vi "nanocal -- nuclear schottky fit V8.vi"() -> ()   [LabVIEW 2021]
uses:
  filename-pattern.ctl
  show-win- control.ctl
  cursor winow.ctl
  nanocal_data_read_format.ctl
  3-lorentzian-parameters.ctl
  nameformattingitem.ctl
  nanocal_side_selector.ctl
  filename-action.ctl
  nanocal -- gradient descent -- parameters.ctl
  linear regression type.ctl
  nanocal-goodness-weighting-strategy.ctl
  3D curvature triplet control -- V2.ctl
  cursor window action.ctl
  cursor action.ctl
  2Dwindow.ctl
  3-lorentzian-heat-response action.ctl
  publisher action.ctl
  <vilib>/Utility/miscctls.llb/LVMapReplaceAction.ctl
  nanocal -- gradient descent -- action.ctl
  array action.ctl
  cursor sate.ctl
  interpolation state - real.ctl
  agregator -- action.ctl
  mathematica string map action.ctl
  nanocal -- defaut parameter manager action-- V1.ctl
  nanocal -- plotstring file action.ctl
  file -- read-write control.ctl
  array -- freq-voltage transformations action.ctl
  nanocal_raw_file_manage_action_V1.ctl
  KM_file -- read-write control.ctl
  replace cursor action stack.vi
  Q -- range multiplier -- real -- V2.vi
  Q - not nan and gtr than zero - Real.vi
  Q - not nan -- real.vi
  Q -- check range -- i -- real.vi
  array - smart min max.vi
  3-lorentzian-heat-response -- V4.vi/142dd4c5-f9ed-c64b-bc14-a88e3e2c450a.vi
  nanocal -- tensors and stuff -- V1.vi
  nanocal -- nuclear schottky goodness V6.vi
  linear interpolation - real -- V2.vi
  <vilib>/AdvancedString/Delimited String to 1D String Array.vi
  array -- freq-voltage transformations.vi/05c44075-957c-bc42-b6fa-2799d0bc0485.vi
  tale of three indices.vi
  filter -- window span logic.vi
  linear interp iiii- complex - z-omega - divide.vi
  linear interpolation iiii- complex.vi
  containing bix.vi
  array -- 3-finitediff.vi
  5-lorentzian-heat-response -- analytic derivatives -- grad and curvature -- V6.vi
  <vilib>/Array/Sort 2D Array - Pop Stack.vi
  <vilib>/Array/Sort 2D Array - Push Stack.vi
  array -- freq-voltage transformations.vi/05c44075-957c-bc42-b6fa-2799d0bc0485.vi/269d4b3b-47f5-49e3-8884-44851e4dd9d5.vi
  array -- freq-voltage transformations.vi/05c44075-957c-bc42-b6fa-2799d0bc0485.vi/6d99389c-673d-4efb-bf33-19b32bcf4cf8.vi
  command stack.vi
  tale of three indices -- check state.vi
  Q -- check range -- i -- integer.vi
  linear interp iiii- complex - z-omega.vi
  line -- complex.vi
  Q - not nan -- integer.vi
  <vilib>/Analysis/baseanly.llb/A x B.vi
  <vilib>/Analysis/baseanly.llb/Complex A x B.vi
  <vilib>/Analysis/Matrix/Numeric/Conversions/Array To Matrix.vi
  <vilib>/Analysis/Matrix/Numeric/Conversions/Array To Matrix - RA2.vi
  <vilib>/Analysis/baseanly.llb/Inverse Matrix.vi
  <vilib>/Analysis/baseanly.llb/Real Inverse Matrix.vi
  <vilib>/Analysis/Matrix/Numeric/Conversions/Matrix To Array.vi
  <vilib>/Analysis/Matrix/Numeric/Conversions/Matrix To Array - RM.vi
  <vilib>/Analysis/Matrix/Numeric/Conversions/Array To Matrix - RA.vi
  <vilib>/Analysis/7linalg.llb/Solve Linear Equations.vi
  <vilib>/Analysis/7linalg.llb/Solve Linear Equations (multiple right hand).vi
  <vilib>/Analysis/polynomials.llb/Polynomial Roots.vi
  <vilib>/Analysis/polynomials.llb/Polynomial Roots (DBL).vi
  <vilib>/Comparison/Less/Less Functor/Less Functor.lvclass
panel:
  in  "tab 8":enum32{"main", "energy profile", "internals"}(tab)
  in  "D. data & fit":enum32{"main"}(tab)
  out "Plot: circles":cluster{"Freq out (Hz)":dbl[], dbl[]}[](graph)
  in  "scale gauge: Plot: circles":dbl(slide)=743510538.726018 min=0.0 max=0.3 step=1e-06 scale=1000000.0..10000000000.0 scale format="%#_3p"
  in  "ω0 (rad/sec)":dbl(slide)=14.871166449464935 scale=0.001..50000.0 scale format="%#_2p"
  in  "E. parameters & open /save":enum32{"logarithmic derivatives"}(tab)
  out "vector of dG/dlogα":dbl[](array[numeric])=[1.7883295749176973, 3.668532274452499, -8.457041272332772, -0.30777115676432043, -0.9594535744754293, -49.05782552987492] format="%#_2f"
  in  "factors":cluster{"scaling":dbl, "what":T1}[](array[cluster])=[{"scaling"=1.0, "what"=enum."ζ"}, {"scaling"=1.0, "what"=enum."τ1"}, {"scaling"=1.0, "what"=enum."τS"}, {"scaling"=1.0, "what"=enum."τN"}, {"scaling"=1.0, "what"=enum."τC"}, {"scaling"=1.0, "what"=enum."κ0"}]
  in  "tab77":enum32{"Page 1"}(tab)
  in  "τC":dbl(slide)=0.001657645209 min=0.0 max=0.3 step=1e-06 scale=0.0001..1.0 scale format="%#_3p"
  in  "τN":dbl(slide)=0.017176281362 min=0.0 max=0.3 step=1e-06 scale=1e-06..1.0 scale format="%#_3p"
  in  "τS":dbl(slide)=0.023837806105 min=0.0 max=0.3 step=1e-06 scale=0.0001..1.0 scale format="%#_3p"
  in  "ζ":dbl(slide)=0.068889386962 min=0.0 max=0.3 step=1e-06 scale=1e-05..1.0 scale format="%#_3p"
  in  "T1":dbl(slide)=0.042189760597 min=0.0 max=0.3 step=1e-06 scale=0.0001..1.0 scale format="%#_3p"
  in  "κ0":dbl(slide)=1.746e-09 min=0.0 max=0.3 step=1e-12 scale=1e-10..1e-06 scale format="%#_3p"
  in  "newton parameters":T2={"method"=enum."newton", "weighting"=enum."dω |dz/dω|", "PID-P"=0.16017985150009284, "PID-I"=3} {"PID-P" scale=1e-09..10.0 scale format="%#_3p"}
  in  "tab 4":enum32{"Page 1"}(tab)
  in  "go / pause!":bool
  in  "tab 7":enum32{"Page 1"}(tab)
  in  "tab 3":enum32{"Page 1"}(tab)
  out "key":string="IDS0187_210310_RAW_cal__ref_"
  out "T (K)":dbl=0.3 format="%#_3f"
  out "θ (deg)":dbl=90.0 format="%#_3f"
  out "B (T)":dbl=12.0 format="%#_3f"
  in  "tab 6":enum32{"Page 1"}(tab)
  in  "τ→Math! :p":bool
  in  "selection :|\\":u16(ring)=5 caption="files" items=["IDS0183_210310_RAW_cal_CeCoIn5_2nd_071_12T_0.120K_90deg_Tdep_raw_.dat", "IDS0184_210310_RAW_cal_CeCoIn5_2nd_072_12T_0.148K_90deg_Tdep_raw_.dat", "IDS0181_210310_RAW_cal_CeCoIn5_2nd_070_12T_0.179K_90deg_fsweep_Tdep_raw_.dat", "IDS0185_210310_RAW_cal_CeCoIn5_2nd_073_12T_0.197K_90deg_Tdep_raw_.dat", "IDS0186_210310_RAW_cal_CeCoIn5_2nd_074_12T_0.249K_90deg_Tdep_raw_.dat", "IDS0187_210310_RAW_cal_CeCoIn5_2nd_075_12T_0.300K_90deg_Tdep_raw_.dat", "IDS0188_210310_RAW_cal_CeCoIn5_2nd_076_12T_0.360K_90deg_Tdep_raw_.dat", "IDS0189_210310_RAW_cal_CeCoIn5_2nd_077_12T_0.430K_90deg_Tdep_raw_.dat", "IDS0190_210310_RAW_cal_CeCoIn5_2nd_078_12T_0.512K_90deg_Tdep_raw_.dat", "IDS0191_210310_RAW_cal_CeCoIn5_2nd_079_12T_0.610K_90deg_Tdep_raw_.dat", "IDS0192_210310_RAW_cal_CeCoIn5_2nd_080_12T_0.810K_90deg_Tdep_raw_.dat", "IDS0193_210310_RAW_cal_CeCoIn5_2nd_081_12T_1.1K_90deg_Tdep_raw_.dat", "IDS0194_210310_RAW_cal_CeCoIn5_2nd_082_12T_1.8K_90deg_Tdep_raw_.dat", "IDS0195_210310_RAW_cal_CeCoIn5_2nd_083_12T_3.0K_90deg_Tdep_raw_.dat", "IDS0196_210310_RAW_cal_CeCoIn5_2nd_084_12T_5.7K_90deg_Tdep_raw_.dat"]
  in  "tab 5":enum32{"Page 1"}(tab)
  in  "Math→τ! :q":bool
  in  "tab 44":enum32{"default values "}(tab)
  in  "defaults selector":T5(array[cluster])=[{"Plost: sweep window"=enum."ζ", "used default"=FALSE}, {"Plost: sweep window"=enum."noiseT", "used default"=TRUE}, {"Plost: sweep window"=enum."τS", "used default"=FALSE}, {"Plost: sweep window"=enum."τN", "used default"=FALSE}, {"Plost: sweep window"=enum."τC", "used default"=FALSE}, {"Plost: sweep window"=enum."Re(offset)", "used default"=TRUE}]
  in  "default values string":string="<| \"0\"->   <|\"T\" -> 0.12, \"Reoff\"-> -130000000.0|>,\n\"1\"->   <|\"T\" -> 0.15, \"Reoff\"-> -70000000.0|>,\n\"2\"->   <|\"T\" -> 0.17, \"Reoff\"-> -50000000.0|>,\n\"3\"->   <|\"T\" -> 0.20, \"Reoff\"-> -28000000.0|>,\n\"4\"->   <|\"T\" -> 0.25, \"Reoff\"-> -14000000.0|>,\n\"5\"->   <|\"T\" -> 0.30, \"Reoff\"-> -8000000.0|>,\n\"6\"->   <|\"T\" -> 0.36, \"Reoff\"-> -4500000.0|>,\n\"7\"->   <|\"T\" -> 0.43, \"Reoff\"-> -3000000.0|>,\n\"8\"->   <|\"T\" -> 0.51, \"Reoff\"-> -2500000.0|>,\n\"9\"->   <|\"T\" -> 0.61, \"Reoff\"-> -1000000.0|>,\n\"10\"->  <|\"T\" -> 0.81, \"Reoff\"-> -700000.0|>,\n\"11\"->  <|\"T\" -> 1.1, \"Reoff\"-> -600000.0|>,\n\"12\"->  <|\"T\" -> 1.8, \"Reoff\"-> -250000.0|>,\n\"13\"->  <|\"T\" -> 3.0, \"Reoff\"-> -130000.0|>,\n\"14\"->  <|\"T\" -> 5.7, \"Reoff\"-> -50000.0|>\n|>\n"
  in  "load defaults":bool
  in  "F. plots & stuff":enum32{"Page 1"}(tab)
  in  "X selector":T1=enum."T (K)"
  in  "Plot:  colors":cluster{"Freq out (Hz)":dbl[], dbl[]}[](graph)=[{"Freq out (Hz)"=[0.12, 0.148, 0.179, 0.197, 0.249, 0.3, 0.36, 0.43, 0.512, 0.61, 0.81, 1.1, 1.8, 3.0, 5.7], [0.375235391174, 0.267189614091, 0.199306617611, 0.169435500052, 0.10023219366, 0.068889386962, 0.050855621628, 0.038379394547, 0.030757711173, 0.024472356387, 0.019125590894, 0.016340595254, 0.01263439258, 0.019026086981, 0.019858524497]}, {"Freq out (Hz)"=[0.12, 0.148, 0.179, 0.197, 0.249, 0.3, 0.36, 0.43, 0.512, 0.61, 0.81, 1.1, 1.8, 3.0, 5.7], [0.100390183494, 0.086925369127, 0.070107577087, 0.06552222252, 0.0499817149, 0.042189760597, 0.035114064267, 0.030049345911, 0.024931554661, 0.022407083343, 0.016432131318, 0.01691523202, 0.012311180561, 0.018297259133, 0.012821278093]}, {"Freq out (Hz)"=[0.12, 0.148, 0.179, 0.197, 0.249, 0.3, 0.36, 0.43, 0.512, 0.61, 0.81, 1.1, 1.8, 3.0, 5.7], [0.059883674441, 0.044416499058, 0.034354681127, 0.031885966152, 0.026964705596, 0.023837806105, 0.021745076003, 0.020197203084, 0.019059366283, 0.017600386438, 0.016139955363, 0.015114072822, 0.011880374999, 0.007367031681, 0.004631070276]}, {"Freq out (Hz)"=[0.12, 0.148, 0.179, 0.197, 0.249, 0.3, 0.36, 0.43, 0.512, 0.61, 0.81, 1.1, 1.8, 3.0, 5.7], [0.583268417564, 0.254096954422, 0.115326183519, 0.085736532349, 0.034498560244, 0.017176281362, 0.009940720882, 0.005279271749, 0.002804912424, 0.001730254025, 0.000695948251, 0.000265648688, 6.6834392e-05, 1.2328467e-05, 1.621029e-06]}, {"Freq out (Hz)"=[0.12, 0.148, 0.179, 0.197, 0.249, 0.3, 0.36, 0.43, 0.512, 0.61, 0.81, 1.1, 1.8, 3.0, 5.7], [0.00101538821, 0.000963914391, 0.001029913549, 0.00108551185, 0.001422553924, 0.001657645209, 0.002035754152, 0.002296433055, 0.00240095569, 0.003444856237, 0.003787605771, 0.003610389555, 0.00409358538, 0.005085235141, 0.003887972994]}, {"Freq out (Hz)"=[], [0.12, 0.13, 0.14, 0.15000000000000002, 0.16000000000000003, 0.17000000000000004, 0.18000000000000005, 0.19000000000000006, 0.20000000000000007, 0.21000000000000008, 0.22000000000000008, 0.2300000000000001, 0.2400000000000001, 0.2500000000000001, 0.2600000000000001, 0.27000000000000013, 0.28000000000000014, 0.29000000000000015, 0.30000000000000016, 0.31000000000000016, 0.3200000000000002, 0.3300000000000002, 0.3400000000000002, 0.3500000000000002, 0.3600000000000002, 0.3700000000000002, 0.3800000000000002, 0.39000000000000024, 0.40000000000000024, 0.41000000000000025, 0.42000000000000026, 0.43000000000000027, 0.4400000000000003, 0.4500000000000003, 0.4600000000000003, 0.4700000000000003, 0.4800000000000003, 0.4900000000000003, 0.5000000000000003, 0.5100000000000003, 0.5200000000000004, 0.5300000000000004, 0.5400000000000004, 0.5500000000000004, 0.5600000000000004, 0.5700000000000004, 0.5800000000000004, 0.5900000000000004, 0.6000000000000004, 0.6100000000000004, 0.6200000000000004, 0.6300000000000004, 0.6400000000000005, 0.6500000000000005, 0.6600000000000005, 0.6700000000000005, 0.6800000000000005, 0.6900000000000005, 0.7000000000000005, 0.7100000000000005, 0.7200000000000005, 0.7300000000000005, 0.7400000000000005, 0.7500000000000006, 0.7600000000000006, 0.7700000000000006, 0.7800000000000006, 0.7900000000000006, 0.8000000000000006, 0.8100000000000006, 0.8200000000000006, 0.8300000000000006, 0.8400000000000006, 0.8500000000000006, 0.8600000000000007, 0.8700000000000007, 0.8800000000000007, 0.8900000000000007, 0.9000000000000007, 0.9100000000000007, 0.9200000000000007, 0.9300000000000007, 0.9400000000000007, 0.9500000000000007, 0.9600000000000007, 0.9700000000000008, 0.9800000000000008, 0.9900000000000008, 1.0000000000000009, 1.0100000000000007, 1.020000000000001, 1.0300000000000007, 1.040000000000001, 1.0500000000000007, 1.060000000000001, 1.0700000000000007, 1.080000000000001, 1.0900000000000007, 1.100000000000001, 1.1100000000000008, 1.120000000000001, 1.1300000000000008, 1.140000000000001, 1.1500000000000008, 1.160000000000001, 1.1700000000000008, 1.180000000000001, 1.1900000000000008, 1.200000000000001, 1.2100000000000009, 1.220000000000001, 1.2300000000000009, 1.240000000000001, 1.2500000000000009, 1.2600000000000011, 1.270000000000001, 1.2800000000000011, 1.290000000000001, 1.3000000000000012, 1.310000000000001, 1.3200000000000012, 1.330000000000001, 1.3400000000000012, 1.350000000000001, 1.3600000000000012, 1.370000000000001, 1.3800000000000012, 1.390000000000001, 1.4000000000000012, 1.410000000000001, 1.4200000000000013, 1.430000000000001, 1.4400000000000013, 1.450000000000001, 1.4600000000000013, 1.470000000000001, 1.4800000000000013, 1.490000000000001, 1.5000000000000013, 1.5100000000000011, 1.5200000000000014, 1.5300000000000011, 1.5400000000000014, 1.5500000000000012, 1.5600000000000014, 1.5700000000000012, 1.5800000000000014, 1.5900000000000012, 1.6000000000000014, 1.6100000000000012, 1.6200000000000014, 1.6300000000000012, 1.6400000000000015, 1.6500000000000012, 1.6600000000000015, 1.6700000000000013, 1.6800000000000015, 1.6900000000000013, 1.7000000000000015, 1.7100000000000013, 1.7200000000000015, 1.7300000000000013, 1.7400000000000015, 1.7500000000000013, 1.7600000000000016, 1.7700000000000014, 1.7800000000000016, 1.7900000000000014, 1.8000000000000016, 1.8100000000000014, 1.8200000000000016, 1.8300000000000014, 1.8400000000000016, 1.8500000000000014, 1.8600000000000017, 1.8700000000000014, 1.8800000000000017, 1.8900000000000015, 1.9000000000000017, 1.9100000000000015, 1.9200000000000017, 1.9300000000000015, 1.9400000000000017, 1.9500000000000015, 1.9600000000000017, 1.9700000000000015, 1.9800000000000018, 1.9900000000000015, 2.0000000000000018, 2.0100000000000016, 2.020000000000002, 2.0300000000000016, 2.040000000000002, 2.0500000000000016, 2.060000000000002, 2.0700000000000016, 2.080000000000002, 2.0900000000000016, 2.100000000000002, 2.1100000000000017, 2.120000000000002, 2.1300000000000017, 2.140000000000002, 2.150000000000002, 2.160000000000002, 2.1700000000000017, 2.180000000000002, 2.190000000000002, 2.200000000000002, 2.2100000000000017, 2.220000000000002, 2.230000000000002, 2.240000000000002, 2.2500000000000018, 2.260000000000002, 2.2700000000000022, 2.280000000000002, 2.290000000000002, 2.300000000000002, 2.3100000000000023, 2.320000000000002, 2.330000000000002, 2.340000000000002, 2.3500000000000023, 2.360000000000002, 2.370000000000002, 2.380000000000002, 2.3900000000000023, 2.400000000000002, 2.410000000000002, 2.420000000000002, 2.4300000000000024, 2.440000000000002, 2.450000000000002, 2.460000000000002, 2.4700000000000024, 2.480000000000002, 2.490000000000002, 2.500000000000002, 2.5100000000000025, 2.5200000000000022, 2.530000000000002, 2.5400000000000023, 2.5500000000000025, 2.5600000000000023, 2.570000000000002, 2.5800000000000023, 2.5900000000000025, 2.6000000000000023, 2.610000000000002, 2.6200000000000023, 2.6300000000000026, 2.6400000000000023, 2.650000000000002, 2.6600000000000024, 2.6700000000000026, 2.6800000000000024, 2.690000000000002, 2.7000000000000024, 2.7100000000000026, 2.7200000000000024, 2.730000000000002, 2.7400000000000024, 2.7500000000000027, 2.7600000000000025, 2.7700000000000022, 2.7800000000000025, 2.7900000000000027, 2.8000000000000025, 2.8100000000000023, 2.8200000000000025, 2.8300000000000027, 2.8400000000000025, 2.8500000000000023, 2.8600000000000025, 2.8700000000000028, 2.8800000000000026, 2.8900000000000023, 2.9000000000000026, 2.910000000000003, 2.9200000000000026, 2.9300000000000024, 2.9400000000000026, 2.950000000000003, 2.9600000000000026, 2.9700000000000024, 2.9800000000000026, 2.990000000000003, 3.0000000000000027, 3.0100000000000025, 3.0200000000000027, 3.030000000000003, 3.0400000000000027, 3.0500000000000025, 3.0600000000000027, 3.070000000000003, 3.0800000000000027, 3.0900000000000025, 3.1000000000000028, 3.110000000000003, 3.1200000000000028, 3.1300000000000026, 3.140000000000003, 3.150000000000003, 3.160000000000003, 3.1700000000000026, 3.180000000000003, 3.190000000000003, 3.200000000000003, 3.2100000000000026, 3.220000000000003, 3.230000000000003, 3.240000000000003, 3.2500000000000027, 3.260000000000003, 3.270000000000003, 3.280000000000003, 3.2900000000000027, 3.300000000000003, 3.310000000000003, 3.320000000000003, 3.3300000000000027, 3.340000000000003, 3.350000000000003, 3.360000000000003, 3.3700000000000028, 3.380000000000003, 3.3900000000000032, 3.400000000000003, 3.410000000000003, 3.420000000000003, 3.4300000000000033, 3.440000000000003, 3.450000000000003, 3.460000000000003, 3.4700000000000033, 3.480000000000003, 3.490000000000003, 3.500000000000003, 3.5100000000000033, 3.520000000000003, 3.530000000000003, 3.540000000000003, 3.5500000000000034, 3.560000000000003, 3.570000000000003, 3.580000000000003, 3.5900000000000034, 3.600000000000003, 3.610000000000003, 3.620000000000003, 3.6300000000000034, 3.6400000000000032, 3.650000000000003, 3.6600000000000033, 3.6700000000000035, 3.6800000000000033, 3.690000000000003, 3.7000000000000033, 3.7100000000000035, 3.7200000000000033, 3.730000000000003, 3.7400000000000033, 3.7500000000000036, 3.7600000000000033, 3.770000000000003, 3.7800000000000034, 3.7900000000000036, 3.8000000000000034, 3.810000000000003, 3.8200000000000034, 3.8300000000000036, 3.8400000000000034, 3.850000000000003, 3.8600000000000034, 3.8700000000000037, 3.8800000000000034, 3.8900000000000032, 3.9000000000000035, 3.9100000000000037, 3.9200000000000035, 3.9300000000000033, 3.9400000000000035, 3.9500000000000037, 3.9600000000000035, 3.9700000000000033, 3.9800000000000035, 3.9900000000000038, 4.0000000000000036, 4.010000000000003, 4.020000000000003, 4.030000000000004, 4.040000000000004, 4.050000000000003, 4.060000000000003, 4.070000000000004, 4.080000000000004, 4.090000000000003, 4.100000000000003, 4.110000000000004, 4.120000000000004, 4.1300000000000034, 4.140000000000003, 4.150000000000004, 4.160000000000004, 4.1700000000000035, 4.180000000000004, 4.190000000000004, 4.200000000000004, 4.2100000000000035, 4.220000000000003, 4.230000000000004, 4.240000000000004, 4.2500000000000036, 4.260000000000004, 4.270000000000004, 4.280000000000004, 4.290000000000004, 4.300000000000003, 4.310000000000004, 4.320000000000004, 4.330000000000004, 4.340000000000004, 4.350000000000004, 4.360000000000004, 4.370000000000004, 4.3800000000000034, 4.390000000000004, 4.400000000000004, 4.410000000000004, 4.420000000000004, 4.430000000000004, 4.440000000000004, 4.450000000000004, 4.4600000000000035, 4.470000000000004, 4.480000000000004, 4.490000000000004, 4.500000000000004, 4.510000000000004, 4.520000000000004, 4.530000000000004, 4.540000000000004, 4.550000000000004, 4.560000000000004, 4.570000000000004, 4.5800000000000045, 4.590000000000004, 4.600000000000004, 4.610000000000004, 4.620000000000004, 4.630000000000004, 4.640000000000004, 4.650000000000004, 4.660000000000005, 4.670000000000004, 4.680000000000004, 4.690000000000004, 4.700000000000004, 4.710000000000004, 4.720000000000004, 4.730000000000004, 4.740000000000005, 4.750000000000004, 4.760000000000004, 4.770000000000004, 4.780000000000004, 4.7900000000000045, 4.800000000000004, 4.810000000000004, 4.820000000000005, 4.8300000000000045, 4.840000000000004, 4.850000000000004, 4.860000000000004, 4.8700000000000045, 4.880000000000004, 4.890000000000004, 4.900000000000005, 4.910000000000005, 4.920000000000004, 4.930000000000004, 4.940000000000004, 4.950000000000005, 4.960000000000004, 4.970000000000004, 4.980000000000005, 4.990000000000005, 5.000000000000004, 5.010000000000004, 5.020000000000004, 5.030000000000005, 5.0400000000000045, 5.050000000000004, 5.060000000000005, 5.070000000000005, 5.0800000000000045, 5.090000000000004, 5.100000000000004, 5.110000000000005, 5.1200000000000045, 5.130000000000004, 5.140000000000005, 5.150000000000005, 5.160000000000005, 5.170000000000004, 5.180000000000004, 5.190000000000005, 5.200000000000005, 5.210000000000004, 5.220000000000005, 5.230000000000005, 5.240000000000005, 5.250000000000004, 5.260000000000004, 5.270000000000005, 5.280000000000005, 5.2900000000000045, 5.300000000000005, 5.310000000000005, 5.320000000000005, 5.3300000000000045, 5.340000000000004, 5.350000000000005, 5.360000000000005, 5.3700000000000045, 5.380000000000005, 5.390000000000005, 5.400000000000005, 5.410000000000005, 5.420000000000004, 5.430000000000005, 5.440000000000005, 5.450000000000005, 5.460000000000005, 5.470000000000005, 5.480000000000005, 5.490000000000005, 5.500000000000004, 5.510000000000005, 5.520000000000005, 5.530000000000005, 5.540000000000005, 5.550000000000005, 5.560000000000005, 5.570000000000005, 5.5800000000000045, 5.590000000000005, 5.600000000000005, 5.610000000000005, 5.620000000000005, 5.630000000000005, 5.640000000000005, 5.650000000000005, 5.660000000000005, 5.670000000000005, 5.680000000000005, 5.690000000000005]}]
  in  "what?":T6={"ignore set of !"=TRUE, "set (1T|2B)"=0, "ignore side !"=FALSE, "side (8S|4R)"=0, "ignore θ !"=FALSE, "ignore B !"=FALSE, "T (K)"=1.0, "ignore T !"=TRUE, "θ (∘)"=4.0, "B (T)"=11.0, "lookup"={"set of lookup"={0=1.0, 1=2.0}, "all set of"={1.0, 2.0}, "T lookup"={0=0.12, 1=0.122, 2=0.14, 3=0.148, 4=0.15, 5=0.157, 6=0.16, 7=0.168, 8=0.17, 9=0.178, 10=0.179, 11=0.18, 12=0.19, 13=0.197, 14=0.2, 15=0.249, 16=0.25, 17=0.255, 18=0.26, 19=0.3, 20=0.307, 21=0.308, 22=0.31, 23=0.36, 24=0.42, 25=0.43, 26=0.438, 27=0.512, 28=0.52, 29=0.53, 30=0.61, 31=0.62, 32=0.63, 33=0.677, 34=0.81, 35=0.82, 36=0.83, 37=1.0, 38=1.1, 39=1.12, 40=1.13, 41=1.25, 42=1.28, 43=1.31, 44=1.39, 45=1.5, 46=1.52, 47=1.55, 48=1.6, 49=1.7, 50=1.8, 51=1.9, 52=2.1, 53=2.3, 54=3.0, 55=3.07, 56=3.1, 57=3.11, 58=5.5, 59=5.7, 60=5.75}, "θ lookup"={0=0.0, 1=30.0, 2=45.0, 3=60.0, 4=90.0}, "B lookup"={0=0.0, 1=1.0, 2=2.0, 3=4.0, 4=5.0, 5=6.0, 6=7.0, 7=8.0, 8=9.0, 9=10.0, 10=11.0, 11=12.0}, "all T's"={0.12, 0.122, 0.14, 0.148, 0.15, 0.157, 0.16, 0.168, 0.17, 0.178, 0.179, 0.18, 0.19, 0.197, 0.2, 0.249, 0.25, 0.255, 0.26, 0.3, 0.307, 0.308, 0.31, 0.36, 0.42, 0.43, 0.438, 0.512, 0.52, 0.53, 0.61, 0.62, 0.63, 0.677, 0.81, 0.82, 0.83, 1.0, 1.1, 1.12, 1.13, 1.25, 1.28, 1.31, 1.39, 1.5, 1.52, 1.55, 1.6, 1.7, 1.8, 1.9, 2.1, 2.3, 3.0, 3.07, 3.1, 3.11, 5.5, 5.7, 5.75}, "all θ's"={0.0, 30.0, 45.0, 60.0, 90.0}, "all B's"={0.0, 1.0, 2.0, 4.0, 5.0, 6.0, 7.0, 8.0, 9.0, 10.0, 11.0, 12.0}, "all sides"={4000.0, 8000.0}, "side lookup"={0=4000.0, 1=8000.0}}} {"B (T)" items=["0.000", "1.000", "2.000", "4.000", "5.000", "6.000", "7.000", "8.000", "9.000", "10.000", "11.000", "12.000"]; "θ (∘)" items=["0.000", "30.000", "45.000", "60.000", "90.000"]; "T (K)" items=["0.120", "0.122", "0.140", "0.148", "0.150", "0.157", "0.160", "0.168", "0.170", "0.178", "0.179", "0.180", "0.190", "0.197", "0.200", "0.249", "0.250", "0.255", "0.260", "0.300", "0.307", "0.308", "0.310", "0.360", "0.420", "0.430", "0.438", "0.512", "0.520", "0.530", "0.610", "0.620", "0.630", "0.677", "0.810", "0.820", "0.830", "1.000", "1.100", "1.120", "1.130", "1.250", "1.280", "1.310", "1.390", "1.500", "1.520", "1.550", "1.600", "1.700", "1.800", "1.900", "2.100", "2.300", "3.000", "3.070", "3.100", "3.110", "5.500", "5.700", "5.750"]; "side (8S|4R)" items=["4000", "8000"]; "set (1T|2B)" items=["1", "2"]}
  in  "colors":enum32{"Page 1"}(tab)
  in  "colors":u32[](array[colorbox])=[7087058, 56538, 2062078, 16740827, 16755712, 11121611, 8285330, 9272482, 9204890]
  in  "parameter list":T1[](array[typedef])=[enum."ζ", enum."τ1", enum."τS", enum."τN", enum."τC", enum."κ0"]
  in  "C. monitor gradient descent":enum32{"main", "more", "file", "notes"}(tab)
  in  "gradient descent monitor tab":enum32{"Page 2"}(tab)
  out "|dln G/dln α_i |":dbl(slide)=49.95861606134944 scale=1e-06..1.0 scale format="%#_3p"
  out "Goodness":dbl(slide)=7.450078630728002e-05 scale=1e-06..1.0 scale format="%#_3p"
  in  "update rate":i32=10
  in  "total # steps":i32=50000
  out "|v_i| = | dG/dlogα_i":dbl[](array[slide])=[1.7883295749176973, 3.668532274452499, 8.457041272332772, 0.30777115676432043, 0.9594535744754293, 49.05782552987492] scale=1e-08..10.0 scale format="%#_2p"
  in  "goodness":enum32{"Page 2", "Page 3"}(tab)
  in  "tab 9":enum32{"Page 1"}(tab)
  in  "#show steps":i32=200
  out "Plot: oscillations":cluster{"Array":i32[], "Array":dbl[]}(graph)={"Array"=[0, 1, 2, 3, 4, 5, 6, 7, 8, 9, 10, 11, 12, 13, 14, 15, 16, 17, 18, 19, 20, 21, 22, 23, 24, 25, 26, 27, 28, 29, 30, 31, 32, 33, 34, 35, 36, 37, 38, 39, 40, 41, 42, 43, 44, 45, 46, 47, 48, 49, 50, 51, 52, 53, 54, 55, 56, 57, 58, 59, 60, 61, 62, 63, 64, 65, 66, 67, 68, 69, 70, 71, 72, 73, 74, 75, 76, 77, 78, 79, 80, 81, 82, 83, 84, 85, 86, 87, 88, 89, 90, 91, 92, 93, 94, 95, 96, 97, 98, 99, 100, 101, 102, 103, 104, 105, 106, 107, 108, 109, 110, 111, 112, 113, 114, 115, 116, 117, 118, 119, 120, 121, 122, 123, 124, 125, 126, 127, 128, 129, 130, 131, 132, 133, 134, 135, 136, 137, 138, 139, 140, 141, 142, 143, 144, 145, 146, 147, 148, 149, 150, 151, 152, 153, 154, 155, 156, 157, 158, 159, 160, 161, 162, 163, 164, 165, 166, 167, 168, 169, 170, 171, 172, 173, 174, 175, 176, 177, 178, 179, 180, 181, 182, 183, 184, 185, 186, 187, 188, 189, 190, 191, 192, 193, 194, 195, 196, 197, 198, 199], "Array"=[-1.7089276453981098e-06, -1.717448211559702e-06, -1.726404714204007e-06, -1.7361822731700393e-06, -1.7469721285025947e-06, -1.758841170501125e-06, -1.771779125118013e-06, -1.785730239499861e-06, -1.800614264542324e-06, -1.816340088625851e-06, -1.8328143616672989e-06, -1.8499467350400838e-06, -1.8676528428665864e-06, -1.8858557996981155e-06, -1.9044867451223986e-06, -1.9234847954782046e-06, -1.942796644720463e-06, -1.962375974874002e-06, -1.982182780449395e-06, -2.0021826730098826e-06, -2.0223462061691086e-06, -2.0426482441409342e-06, -2.0630673855136293e-06, -2.083585446673508e-06, -2.1041870047600443e-06, -2.124858997251851e-06, -2.1455903739183184e-06, -2.1663717960902318e-06, -2.1871953780677397e-06, -2.208054465699166e-06, -2.228943447253433e-06, -2.249857592411485e-06, -2.270792915474182e-06, -2.291746059256009e-06, -2.3127141968193343e-06, -2.33369494827344e-06, -2.354686310485695e-06, -2.375686597752547e-06, -2.3966943916521382e-06, -2.417708498853987e-06, -2.4387279154762195e-06, -2.4597517970997916e-06, -2.4807794334588185e-06, -2.5018102272059335e-06, -2.52284367594516e-06, -2.543879357189854e-06, -2.5649169156465295e-06, -2.5859560525323786e-06, -2.6069965166224704e-06, -2.6280380966561627e-06, -2.6490806149917544e-06, -2.6701239222606094e-06, -2.6911678928737896e-06, -2.712212421223444e-06, -2.7332574185157457e-06, -2.754302810091991e-06, -2.7753485331852225e-06, -2.796394535007913e-06, -2.817440771185945e-06, -2.838487204404115e-06, -2.859533803296671e-06, -2.8805805414760296e-06, -2.9016273967707984e-06, -2.9226743505348144e-06, -2.943721387088671e-06, -2.9647684932560046e-06, -2.985815657939627e-06, -3.006862871839794e-06, -3.0279101271053635e-06, -3.048957417155717e-06, -3.0700047364608804e-06, -3.0910520803441484e-06, -3.1120994449085186e-06, -3.1331468268551432e-06, -3.1541942234135064e-06, -3.1752416322618974e-06, -3.1962890514430605e-06, -3.217336479308412e-06, -3.2383839144784128e-06, -3.2594313557890637e-06, -3.280478802261818e-06, -3.3015262530747963e-06, -3.3225737075460353e-06, -3.343621165073532e-06, -3.3646686251814295e-06, -3.385716087465538e-06, -3.4067635515733826e-06, -3.4278110172104945e-06, -3.4488584841379155e-06, -3.4699059521481833e-06, -3.4909534210714036e-06, -3.512000890762781e-06, -3.5330483610951932e-06, -3.554095831969598e-06, -3.5751433032999097e-06, -3.59619077501121e-06, -3.6172382470476085e-06, -3.638285719356196e-06, -3.659333191886286e-06, -3.6803806646103937e-06, -3.7014281374988123e-06, -3.7224756105186906e-06, -3.7435230836563673e-06, -3.764570556883274e-06, -3.785618030197242e-06, -3.806665503573606e-06, -3.82771297701307e-06, -3.84876045049303e-06, -3.869807924014514e-06, 0.00018389091337609896, 0.00013689095914755828, 8.702754364029748e-05, 5.973666657432358e-05, 4.100781302927717e-05, 2.7669973614823605e-05, 1.8287977055077764e-05, 1.1716873713820146e-05, 7.124468923382608e-06, 3.9239030368697515e-06, 1.700764014506324e-06, 1.62438368951222e-07, -8.973652858690188e-07, -1.623840618003396e-06, -2.1189973140014117e-06, -2.4543597697744514e-06, -2.679959230666583e-06, -2.8306949245066634e-06, -2.9308293804979828e-06, -2.99716182388277e-06, -3.041265835989303e-06, -3.071065229607521e-06, -3.0919423028046207e-06, -3.107515975118015e-06, -3.120187109891448e-06, -3.131519827558678e-06, -3.14250742479064e-06, -3.153757221141789e-06, -3.1656185427770167e-06, -3.1782709029518205e-06, -3.191784387537118e-06, -3.206160687185247e-06, -3.221360701262941e-06, -3.23732286547151e-06, -3.2539751054456523e-06, -3.2712424407873924e-06, -3.2890516464371424e-06, -3.3073339458014324e-06, -3.3260264071384134e-06, -3.345072503048571e-06, -3.364422145919028e-06, -3.384031409708432e-06, -3.403862077916832e-06, -3.42388110917836e-06, -3.4440600786024827e-06, -3.464374630634409e-06, -3.4848039642207678e-06, -3.505330361172447e-06, -3.5259387620313718e-06, -3.546616390098572e-06, -3.567352421459096e-06, -3.5881376978125234e-06, -3.608964478110058e-06, -3.6298262248049377e-06, -3.6507174206859626e-06, -3.6716334124052216e-06, -3.6925702771886085e-06, -3.713524709503626e-06, -3.7344939249384134e-06, -3.755475578714248e-06, -3.7764676967835765e-06, -3.7974686175523058e-06, -3.818476942657348e-06, -3.839491495465205e-06, -3.860511286011474e-06, -3.881535481495041e-06, -3.902563381363822e-06, -3.923594396393782e-06, -3.944628030991227e-06, -3.965663868358811e-06, -3.986701557979013e-06, -4.0077408050759105e-06, -4.028781361774974e-06, -4.049823019630638e-06, -4.0708656033793455e-06, -4.091908965623756e-06, -4.112952982441296e-06, -4.133997549625608e-06, -4.155042579570827e-06, -4.176087998595439e-06, -4.1971337447539335e-06, -4.2181797659717e-06, -4.239226018453151e-06, -4.260272465382955e-06, -4.281319075797056e-06, -4.302365823666851e-06, -4.323412687104412e-06, -4.344459647715219e-06, -4.365506690029333e-06, -4.386553801031992e-06, -4.4076009697894495e-06]}
  out "current step":i32=92
  out "update  ind":i32=18
  in  "generate empty string from filelist !":bool
  in  "toggle generate labview files":bool
  in  "data file formatting":T7=enum."raw nanocal"
  in  "save data":enum32{"save/read"}(tab)
  in  "Save to file :s":bool
  in  "Freq sweep name template":T8={"prefix"="RuCl3-rod", "group"="f"}
  in  "Save folder":path=path "/opt/data"
  in  "freq sweep file name":string="f013_RuCl3-rod_082821.dat"
  out "correct temperature":dbl min=10.0 max=10000.0 step=10.0
  in  "side":T9=enum."ref"
  in  "string notes":string="\"T\"-> 0.225000,    \"ζ\"-> 0.006057  , \"τ1\"-> 0.011106  , \"τS\"-> 0.134857  , \"τN\"-> 0.000042  , \"τC\"-> 0.012982  , \"κ0\"-> 0.000000101776  , \"mm1\"-> 0.000071  , \"mm2\"-> 0.148631  , \"mm3\"-> 0.011103 "
  in  "load! :l":bool
  in  "Read from file":path=path "/Users/arkadyshekhter/Library/CloudStorage/Dropbox/shared_AkashAndreas/paper-CeCoIn5-spectroheat/Original RAW data/Original RAW files (IDS0110 to IDS0220)/IDS0187_210310_RAW_cal_CeCoIn5_2nd_075_12T_0.300K_90deg_Tdep_raw_.dat"
  in  "parse! :p":bool
  in  "String":string=" <|    \"ζ\" -> 0.068889386962   ,  \"τ1\" -> 0.042189760597   ,  \"τS\" -> 0.023837806105   ,  \"τN\" -> 0.017176281362   ,  \"τC\" -> 0.001657645209   ,  \"κ0\" -> 0.000000001746   ,  \"mm1\" -> 0.000100672139   ,  \"mm2\" -> 0.015917651868   ,  \"mm3\" -> 0.071668604609   ,  \"T\" -> 0.300000000000   ,  \"B\" -> 12.000000000000   ,  \"θ\" -> 90.000000000000   ,  \"Reoff\" -> 0.000000000000   ,  \"Imoff\" -> 0.000000000000   ,  \"στ1\" -> 0.000000000000   ,  \"στS\" -> 0.000000000000   ,  \"στN\" -> 0.000000000000   ,  \"τ11 \" -> 0.000000000000   ,  \"τ12\" -> 0.000000000000   ,  \"τ22\" -> 0.000000000000   ,  \"τN1\" -> 0.000000000000   ,  \"τN2\" -> 0.000000000000   ,  \"σηlogτ1 \" -> 0.000000000000   ,  \"σηlogτS\" -> 0.000000000000   ,  \"σηlogτN\" -> 0.000000000000   ,  \"σlogτ1\" -> 0.000000000000   ,  \"σlogτS\" -> 0.000000000000   ,  \"σlogτN\" -> 0.000000000000   ,  \"σητ1\" -> 0.000000000000   ,  \"σητS \" -> 0.000000000000   ,  \"σητN\" -> 0.000000000000   ,  \"noiseT\" -> 0.000000000000    |> "
  in  "newton is active":bool
  out "file IDS":string="IDS0187_210310_RAW_cal_"
  out "notes":string="------------\n\n/opt/new/Dropbox/desktop_data/Indium-nanocal-cell12-June2021/labview-ready-files\nIndium_June2021_*_ark.dat\n\n---------------------\n/opt/new/Dropbox/shared_AkashAndreas/paper-CeCoIn5/labviewreadydata\nCeCoIn5_*_labview_.dat\n--------------------------------\n\n  48 ->   <| \"ζ\"->  0.219100303741  , \"τ1\"-> 0.028643012604  , \"τS\"-> 0.279362928811  , \"τN\"-> 0.246156444058  , \"τC\"-> 0.001272401549  , \"κ0\"-> 0.000000000760  , \"mm1\"-> 0.000227975653  , \"mm2\"-> 0.014929571562  , \"mm3\"-> 0.655418694024  , \"T\"->  0.148000000000  , \"B\"-> 12.000000000000  , \"θ\"-> 0.000000000000  |>   , \r49 ->   <| \"ζ\"->  0.172530402516  , \"τ1\"-> 0.028151242536  , \"τS\"-> 0.147833386881  , \"τN\"-> 0.151615465647  , \"τC\"-> 0.001078987959  , \"κ0\"-> 0.000000001040  , \"mm1\"-> 0.000157922197  , \"mm2\"-> 0.013374167913  , \"mm3\"-> 0.366811023972  , \"T\"->  0.179000000000  , \"B\"-> 12.000000000000  , \"θ\"-> 0.000000000000  |>   , \r50 ->   <| \"ζ\"->  0.133463068512  , \"τ1\"-> 0.025720252342  , \"τS\"-> 0.123146502099  , \"τN\"-> 0.097478248186  , \"τC\"-> 0.001335222055  , \"κ0\"-> 0.000000001204  , \"mm1\"-> 0.000155896243  , \"mm2\"-> 0.013755191011  , \"mm3\"-> 0.263214393590  , \"T\"->  0.197000000000  , \"B\"-> 12.000000000000  , \"θ\"-> 0.000000000000  |>   , \r51 ->   <| \"ζ\"->  0.081993362741  , \"τ1\"-> 0.028064095915  , \"τS\"-> 0.091433392476  , \"τN\"-> 0.030443971714  , \"τC\"-> 0.001450504959  , \"κ0\"-> 0.000000001536  , \"mm1\"-> 0.000108446090  , \"mm2\"-> 0.019905820843  , \"mm3\"-> 0.141370833064  , \"T\"->  0.250000000000  , \"B\"-> 12.000000000000  , \"θ\"-> 0.000000000000  |>   , \r52 ->   <| \"ζ\"->  0.054088186012  , \"τ1\"-> 0.023838802615  , \"τS\"-> 0.069079396629  , \"τN\"-> 0.016435267456  , \"τC\"-> 0.002025071743  , \"κ0\"-> 0.000000001955  , \"mm1\"-> 0.000101234646  , \"mm2\"-> 0.018244822177  , \"mm3\"-> 0.097657814678  , \"T\"->  0.300000000000  , \"B\"-> 12.000000000000  , \"θ\"-> 0.000000000000  |>   , \r53 ->   <| \"ζ\"->  0.039314966212  , \"τ1\"-> 0.020712803909  , \"τS\"-> 0.055413767550  , \"τN\"-> 0.008474403424  , \"τC\"-> 0.002674063387  , \"κ0\"-> 0.000000002415  , \"mm1\"-> 0.000096818147  , \"mm2\"-> 0.017190811405  , \"mm3\"-> 0.072499170001  , \"T\"->  0.360000000000  , \"B\"-> 12.000000000000  , \"θ\"-> 0.000000000000  |>   , \r54 ->   <| \"ζ\"->  0.031945976845  , \"τ1\"-> 0.019000922826  , \"τS\"-> 0.045624146388  , \"τN\"-> 0.005314716063  , \"τC\"-> 0.002488383471  , \"κ0\"-> 0.000000002954  , \"mm1\"-> 0.000073272643  , \"mm2\"-> 0.016306894362  , \"mm3\"-> 0.057675293464  , \"T\"->  0.430000000000  , \"B\"-> 12.000000000000  , \"θ\"-> 0.000000000000  |>   , \r55 ->   <| \"ζ\"->  0.023031239946  , \"τ1\"-> 0.018268814012  , \"τS\"-> 0.037269400776  , \"τN\"-> 0.002696792890  , \"τC\"-> 0.003257395394  , \"κ0\"-> 0.000000003720  , \"mm1\"-> 0.000067670174  , \"mm2\"-> 0.016445281937  , \"mm3\"-> 0.045899921957  , \"T\"->  0.512000000000  , \"B\"-> 12.000000000000  , \"θ\"-> 0.000000000000  |>   , \r56 ->   <| \"ζ\"->  0.019920170845  , \"τ1\"-> 0.016368892412  , \"τS\"-> 0.030579536580  , \"τN\"-> 0.001736017565  , \"τC\"-> 0.004971418152  , \"κ0\"-> 0.000000004410  , \"mm1\"-> 0.000083939556  , \"mm2\"-> 0.015095997595  , \"mm3\"-> 0.039119658918  , \"T\"->  0.610000000000  , \"B\"-> 12.000000000000  , \"θ\"-> 0.000000000000  |>   , \r57 ->   <| \"ζ\"->  0.017558473054  , \"τ1\"-> 0.014545104284  , \"τS\"-> 0.022979681288  , \"τN\"-> 0.000840829385  , \"τC\"-> 0.005228030240  , \"κ0\"-> 0.000000006068  , \"mm1\"-> 0.000073916527  , \"mm2\"-> 0.013750428362  , \"mm3\"-> 0.030187552103  , \"T\"->  0.810000000000  , \"B\"-> 12.000000000000  , \"θ\"-> 0.000000000000  |>   , \r58 ->   <| \"ζ\"->  0.011916480594  , \"τ1\"-> 0.012551282481  , \"τS\"-> 0.018233218660  , \"τN\"-> 0.000345702746  , \"τC\"-> 0.004699451527  , \"κ0\"-> 0.000000008451  , \"mm1\"-> 0.000044190864  , \"mm2\"-> 0.012162820727  , \"mm3\"-> 0.023844039179  , \"T\"->  1.120000000000  , \"B\"-> 12.000000000000  , \"θ\"-> 0.000000000000  |>   , \r59 ->   <| \"ζ\"->  0.012831327568  , \"τ1\"-> 0.013315909415  , \"τS\"-> 0.012590836847  , \"τN\"-> 0.000065003013  , \"τC\"-> 0.005276356243  , \"κ0\"-> 0.000000013610  , \"mm1\"-> 0.000047406274  , \"mm2\"-> 0.013137605540  , \"mm3\"-> 0.018225484932  , \"T\"->  1.800000000000  , \"B\"-> 12.000000000000  , \"θ\"-> 0.000000000000  |>   , \r60 ->   <| \"ζ\"->  0.019774146838  , \"τ1\"-> 0.013257273421  , \"τS\"-> 0.007064131508  , \"τN\"-> 0.000028000819  , \"τC\"-> 0.006942241845  , \"κ0\"-> 0.000000023477  , \"mm1\"-> 0.000068886863  , \"mm2\"-> 0.012935419574  , \"mm3\"-> 0.014427582022  , \"T\"->  3.000000000000  , \"B\"-> 12.000000000000  , \"θ\"-> 0.000000000000  |>   , \r61 ->   <| \"ζ\"->  0.029251354442  , \"τ1\"-> 0.014634751206  , \"τS\"-> 0.003873958746  , \"τN\"-> 0.000007000487  , \"τC\"-> 0.006827504775  , \"κ0\"-> 0.000000056438  , \"mm1\"-> 0.000072018576  , \"mm2\"-> 0.010723236476  , \"mm3\"-> 0.014661483476  , \"T\"->  5.500000000000  , \"B\"-> 12.000000000000  , \"θ\"-> 0.000000000000  |>   , \r70 ->   <| \"ζ\"->  0.166131699293  , \"τ1\"-> 0.072775930308  , \"τS\"-> 0.042465819987  , \"τN\"-> 0.161702990281  , \"τC\"-> 0.001278548133  , \"κ0\"-> 0.000000001029  , \"mm1\"-> 0.000178150965  , \"mm2\"-> 0.012296129795  , \"mm3\"-> 0.299667919341  , \"T\"->  0.179000000000  , \"B\"-> 12.000000000000  , \"θ\"-> 90.000000000000  |>   , \r71 ->   <| \"ζ\"->  0.300863384227  , \"τ1\"-> 0.104924004009  , \"τS\"-> 0.071070599729  , \"τN\"-> 0.992887187112  , \"τC\"-> 0.001721587800  , \"κ0\"-> 0.000000000548  , \"mm1\"-> 0.000392216822  , \"mm2\"-> 0.006637384427  , \"mm3\"-> 1.483679717825  , \"T\"->  0.120000000000  , \"B\"-> 12.000000000000  , \"θ\"-> 90.000000000000  |>   , \r72 ->   <| \"ζ\"->  0.222191124978  , \"τ1\"-> 0.096157808510  , \"τS\"-> 0.068016409177  , \"τN\"-> 0.365932480375  , \"τC\"-> 0.001342124138  , \"κ0\"-> 0.000000000769  , \"mm1\"-> 0.000240761160  , \"mm2\"-> 0.013184061080  , \"mm3\"-> 0.614443591912  , \"T\"->  0.148000000000  , \"B\"-> 12.000000000000  , \"θ\"-> 90.000000000000  |>   , \r73 ->   <| \"ζ\"->  0.136299067728  , \"τ1\"-> 0.070555788073  , \"τS\"-> 0.041728112583  , \"τN\"-> 0.122673380524  , \"τC\"-> 0.001576035942  , \"κ0\"-> 0.000000001215  , \"mm1\"-> 0.000183611814  , \"mm2\"-> 0.014077355758  , \"mm3\"-> 0.244680119794  , \"T\"->  0.197000000000  , \"B\"-> 12.000000000000  , \"θ\"-> 90.000000000000  |>   , \r74 ->   <| \"ζ\"->  0.083818989463  , \"τ1\"-> 0.054019568165  , \"τS\"-> 0.033709166928  , \"τN\"-> 0.048192327645  , \"τC\"-> 0.001574712191  , \"κ0\"-> 0.000000001532  , \"mm1\"-> 0.000117096712  , \"mm2\"-> 0.016005996433  , \"mm3\"-> 0.128237582295  , \"T\"->  0.249000000000  , \"B\"-> 12.000000000000  , \"θ\"-> 90.000000000000  |>   , \r75 ->   <| \"ζ\"->  0.057938569833  , \"τ1\"-> 0.045244527663  , \"τS\"-> 0.029709028064  , \"τN\"-> 0.023577376257  , \"τC\"-> 0.002006607539  , \"κ0\"-> 0.000000001948  , \"mm1\"-> 0.000103608352  , \"mm2\"-> 0.017542867394  , \"mm3\"-> 0.085978401835  , \"T\"->  0.300000000000  , \"B\"-> 12.000000000000  , \"θ\"-> 90.000000000000  |>   , \r76 ->   <| \"ζ\"->  0.044154556051  , \"τ1\"-> 0.038823125235  , \"τS\"-> 0.027069314930  , \"τN\"-> 0.013601990730  , \"τC\"-> 0.002287979276  , \"κ0\"-> 0.000000002359  , \"mm1\"-> 0.000089763345  , \"mm2\"-> 0.018083678254  , \"mm3\"-> 0.065404792018  , \"T\"->  0.360000000000  , \"B\"-> 12.000000000000  , \"θ\"-> 90.000000000000  |>   , \r77 ->   <| \"ζ\"->  0.032748569996  , \"τ1\"-> 0.031072007290  , \"τS\"-> 0.024343937548  , \"τN\"-> 0.006961654481  , \"τC\"-> 0.002967111565  , \"κ0\"-> 0.000000002964  , \"mm1\"-> 0.000084402249  , \"mm2\"-> 0.018055855929  , \"mm3\"-> 0.048229666078  , \"T\"->  0.430000000000  , \"B\"-> 12.000000000000  , \"θ\"-> 90.000000000000  |>   , \r78 ->   <| \"ζ\"->  0.027599263457  , \"τ1\"-> 0.026239105728  , \"τS\"-> 0.022370859308  , \"τN\"-> 0.003857632966  , \"τC\"-> 0.003499360499  , \"κ0\"-> 0.000000003681  , \"mm1\"-> 0.000081816106  , \"mm2\"-> 0.017901054668  , \"mm3\"-> 0.038707974796  , \"T\"->  0.512000000000  , \"B\"-> 12.000000000000  , \"θ\"-> 90.000000000000  |>   , \r79 ->   <| \"ζ\"->  0.020568815513  , \"τ1\"-> 0.023045965648  , \"τS\"-> 0.020791387386  , \"τN\"-> 0.002229171297  , \"τC\"-> 0.004427475438  , \"κ0\"-> 0.000000004398  , \"mm1\"-> 0.000074037290  , \"mm2\"-> 0.017820522459  , \"mm3\"-> 0.033072945644  , \"T\"->  0.610000000000  , \"B\"-> 12.000000000000  , \"θ\"-> 90.000000000000  |>   , \r80 ->   <| \"ζ\"->  0.016159836955  , \"τ1\"-> 0.019958638777  , \"τS\"-> 0.018730096307  , \"τN\"-> 0.000899236968  , \"τC\"-> 0.005152267403  , \"κ0\"-> 0.000000006087  , \"mm1\"-> 0.000064651231  , \"mm2\"-> 0.017530317649  , \"mm3\"-> 0.027462477400  , \"T\"->  0.810000000000  , \"B\"-> 12.000000000000  , \"θ\"-> 90.000000000000  |>   , \r81 ->   <| \"ζ\"->  0.014495870556  , \"τ1\"-> 0.019990087457  , \"τS\"-> 0.016832201384  , \"τN\"-> 0.000455517238  , \"τC\"-> 0.005555782498  , \"κ0\"-> 0.000000008420  , \"mm1\"-> 0.000060055560  , \"mm2\"-> 0.018114231010  , \"mm3\"-> 0.024909902538  , \"T\"->  1.100000000000  , \"B\"-> 12.000000000000  , \"θ\"-> 90.000000000000  |>   , \r82 ->   <| \"ζ\"->  0.014043763709  , \"τ1\"-> 0.018292068543  , \"τS\"-> 0.011311396743  , \"τN\"-> 0.000128802259  , \"τC\"-> 0.008087849636  , \"κ0\"-> 0.000000014258  , \"mm1\"-> 0.000065912054  , \"mm2\"-> 0.017276417784  , \"mm3\"-> 0.020638450794  , \"T\"->  1.800000000000  , \"B\"-> 12.000000000000  , \"θ\"-> 90.000000000000  |>   , \r83 ->   <| \"ζ\"->  0.016187684631  , \"τ1\"-> 0.018325345271  , \"τS\"-> 0.007510087776  , \"τN\"-> 0.000028419157  , \"τC\"-> 0.008115463080  , \"κ0\"-> 0.000000024747  , \"mm1\"-> 0.000062903858  , \"mm2\"-> 0.015524812312  , \"mm3\"-> 0.018513630087  , \"T\"->  3.000000000000  , \"B\"-> 12.000000000000  , \"θ\"-> 90.000000000000  |>   , \r84 ->   <| \"ζ\"->  0.027897403691  , \"τ1\"-> 0.014639690770  , \"τS\"-> 0.004105291179  , \"τN\"-> 0.000006999171  , \"τC\"-> 0.007414449545  , \"κ0\"-> 0.000000059701  , \"mm1\"-> 0.000073450671  , \"mm2\"-> 0.011534391407  , \"mm3\"-> 0.014673310811  , \"T\"->  5.700000000000  , \"B\"-> 12.000000000000  , \"θ\"-> 90.000000000000  |>   , \r"
  in  "backup string :b":string=" <| \"ζ\"->  0.167234158379  , \"τ1\"-> 0.020665214756  , \"τS\"-> 0.072250691270  , \"τN\"-> 0.020708769022  , \"τC\"-> 0.001243822553  , \"κ0\"-> 0.000000001059  , \"mm1\"-> 0.000000000000  , \"mm2\"-> 0.000000000000  , \"mm3\"-> 0.000000000000  , \"T\"->  5.700000000000  , \"B\"-> 12.000000000000  , \"θ\"-> 45.000000000000  |> "
  in  "B.  errors & stuff":enum32{"Page 1"}(tab) caption="curvature & stuff"
  in  "error weights":T4=enum."anti-andr"
  in  "errors&stuff":T10={"one"=enum."τ1", "two"=enum."τS", "sigmaone"=enum."στ1", "sigmatwo"=enum."στS", "three"=enum."τN", "sigmathree"=enum."στN", "pars & errors"={enum."τ1"=0.042189760597, enum."τS"=0.023837806105, enum."τN"=0.017176281362, enum."στ1"=0.0018935121063218513, enum."στS"=4.1582736953258186e-05, enum."στN"=0.000674370512501787, enum."σηlogτ1"=0.02212459673922192, enum."σηlogτS"=2.839610896625299e-05, enum."σηlogτN"=0.038783672526097525, enum."σlogτ1"=0.04488084500902558, enum."σlogτS"=0.0017444028519275592, enum."σlogτN"=0.03926172949132823, enum."σητ1"=0.0009334314397329396, enum."σητS"=6.769009396739908e-07, enum."σητN"=0.0006661592715599204}, "T22 factor"=5.043159, "CN2 factor"=0.09999999999999998, "δG/G"=0.10291154062341111, "noise T"=0.001, "Δlogs"=[0.04488084500902558, 0.0017444028519275592, 0.03926172949132823], "Δlog ηs"=[0.02212459673922192, 2.839610896625299e-05, 0.038783672526097525]} {"Δlog ηs" format="%#_2f"; "Δlogs" format="%#_2f"; "noise T" format="%#_3f"; "δG/G" format="%#_3f"; "CN2 factor" min=0.0 max=0.3 step=1e-06 scale=0.01..1.0 scale format="%#_2f"; "T22 factor" min=0.0 max=0.3 step=1e-06 scale=0.1..20.0 scale format="%#_2f"}
  in  "update errors as you fit":bool=TRUE
  in  "overwrite noiseT":bool
  in  "A. data load & stuff":enum32{"Page 2"}(tab)
  in  "|ω| < limit (Hz)":dbl(slide)=2520.283192526746 min=10.0 max=10000.0 step=10.0 scale=50.0..5000.0 scale format="%#_3p"
  in  "offset Re\noffset Im":cluster{"Numeric":dbl, "Numeric":dbl}(slide)={"Numeric"=-7999999.999999998, "Numeric"=0.0} scale=-300000000.0..1000000.0 scale format="%#_1p"
  in  "overwrite \noffset":bool=TRUE
